vi "Save Runtime Menu to RTF File.vi"() -> ()   [LabVIEW 2012, in "VIRef.lvlib"]
uses:
  VIRef.lvlib
panel:
  out "错误输出":errorcluster
  in  "错误输入（无错误）":errorcluster
  in  "VI Ref":refnum<vi>
  in  "Menu File Path":path
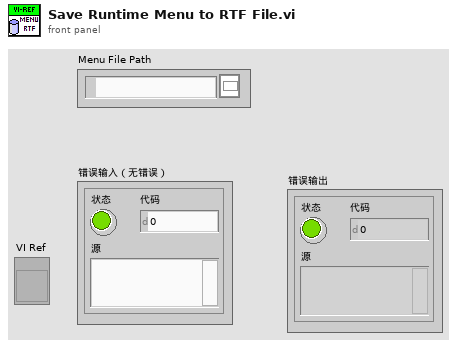
[diagram p1: front panel]
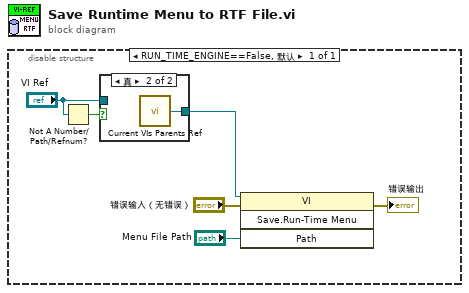
[diagram p0: block diagram]
diagram:
  n1 = disable-structure shown="RUN_TIME_ENGINE==False, 默认" {
    frame condition #0 (active) {
      n2 = Not A Number/Path/Refnum?(number/path/refnum="VI Ref") -> (NaN/Path/Refnum?=w5:bool)
      n3 = case shown="真" w5 {
        tunnel: [w7 w8] -> w3
        tunnel: "VI Ref" -> [w7 _]
        frame False {
        }
        frame True {
          n4 = call "Current VIs Parents Ref.vi"() -> ("Calling VI's Reference"=w8:refnum<vi>)  [unwired: 2 in]
        }
      }
      n5 = invoke class="VI" method="Save.Run-Time Menu"(reference=w3, error in="错误输入（无错误）", "Path"="Menu File Path") -> (error out=→"错误输出":errorcluster)  [unwired: 1 in, 3 out]
    }
  }
